vi "10aread.vi"() -> ()   [LabVIEW 2013]
panel:
  out "size (in bytes)":i64
  out "text":string
  in  "file path (use dialog)":path
  # "G.SURESH\n23A91A0417\nECE-A"
  # "10A) FILE I/O OPERATIONS (READ OPERATION)"
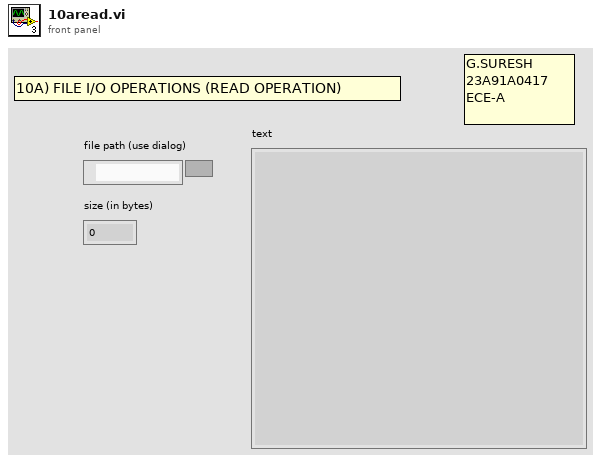
[diagram p1: front panel]
types:
  T1 = enum16{"open", "replace", "create", "open or create", "replace or create", "replace or create with confirmation"}
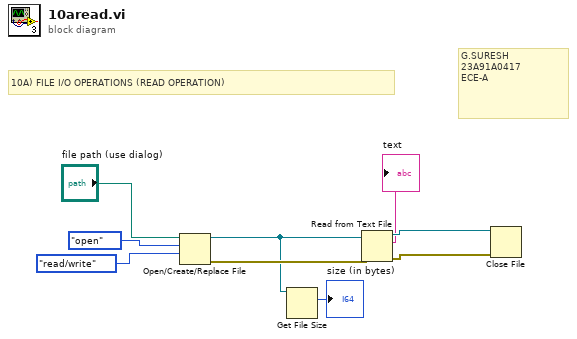
[diagram p0: block diagram]
diagram:
  # "10A) FILE I/O OPERATIONS (READ OPERATION)"
  # "G.SURESH\n23A91A0417\nECE-A"
  n1 = Open/Create/Replace File(file path (use dialog)="file path (use dialog)", operation (0:open)=T1."open", access (0:read/write)=enum16{"read/write", "read-only", "write-only"}."read/write") -> (refnum out=w2:refnum<file>, error out=w8:errorcluster)  [unwired: 3 in, 1 out]
  n2 = Get File Size(file=w2) -> (size (in bytes)=→"size (in bytes)":i64)  [unwired: 1 in, 2 out]
  n3 = Read from Text File(file (use dialog)=w2, error in=w8) -> (refnum out=w9:refnum<file>, text=→"text":string, error out=w7:errorcluster)  [unwired: 2 in, 1 out]
  n4 = Close File(refnum=w9, error in=w7) -> ()  [unwired: 2 out]
